vi "piston manipulation test.vi"() -> (0 "Shooter":T1, 1 "Lock":T1)   [LabVIEW 2013]
uses:
  <vilib>/Rock Robotics/WPI/Solenoid/WPI_SolenoidValue.ctl
  <vilib>/Rock Robotics/WPI/Joystick/WPI_JoystickGetSetRefNum.vi
panel:
  # "Joystick 1button 5 activates lock\njoystick 1 button 3 deactivates lock\njoystick 1 button 6 activates shooter\njoystick 1 button 4 deactivates shooter"
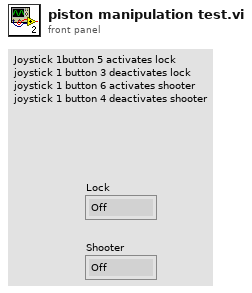
[diagram p1: front panel]
types:
  T1 = typedef "WPI_SolenoidValue.ctl" = enum16{"Off", "On", "Forward", "Reverse"}
  T2 = typedef "WPI_JoystickDevRef.ctl" = cluster{"Device":T3}
  T3 = typedef "WPI_JoystickDeviceEnum.ctl" = enum16{"USB 1", "USB 2", "USB 3", "USB 4", "Kinect 1", "Kinect 2"}
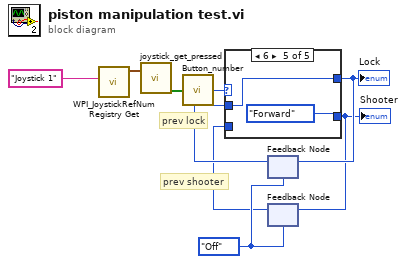
[diagram p0: block diagram]
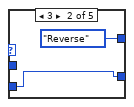
[diagram p3: hidden frame]
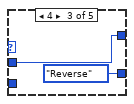
[diagram p4: hidden frame]
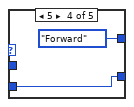
[diagram p5: hidden frame]
diagram:
  w5 = WPI_SolenoidValue."Off" ("Value")
  # "prev lock"
  # "prev shooter"
  n1 = call <vilib>:"WPI_JoystickRefNum Registry Get.vi"("refnum name"="Joystick 1") -> ("JoystickDevRef"=w9:T2)  [unwired: 9 in, 1 out]
  n2 = call "joystick_get_pressed.vi"("JoystickDevRef 2"=w9) -> ("Buttons Pressed?"=w7:bool[])  [unwired: 1 in, 3 out]
  n3 = call "Button_number.vi"("Button Array"=w7) -> ("Button Pressed"=w6:i32)
  n4 = feedback #1(w5) -> (w2:T1)
  n5 = feedback #2(w5) -> (w1:T1)
  n6 = case shown="6" w6 {
    tunnel: [w11 WPI_SolenoidValue."Reverse" ("Value") w15 WPI_SolenoidValue."Forward" ("Value") w18] -> w4
    tunnel: [w10 w12 WPI_SolenoidValue."Reverse" ("Value") w16 WPI_SolenoidValue."Forward" ("Value")] -> w3
    tunnel: w2 -> [w11 _ w15 _ w18]
    tunnel: w1 -> [w10 w12 _ w16 _]
    frame 0, Default {
    }
    frame 3 {
    }
    frame 4 {
    }
    frame 5 {
    }
    frame 6 {
    }
  }
  "Lock" <- w4
  "Shooter" <- w3
  n7 = feedback-in #1(w4) -> ()
  n8 = feedback-in #2(w3) -> ()
